vi "Set Description.vi"(8 "error in":errorcluster, 10 "description":string, 11 "data sharing framework custom device in":T1 format="%.0x") -> (0 "error out":errorcluster, 3 "data sharing framework custom deviceout":T1 format="%.0x")   [LabVIEW 2017, in "Data Sharing Framework Custom Device Scripting.lvlib"]
doc: "Writes the <b>description</b> field for the input Data Sharing Framework custom device."
uses:
  Data Sharing Framework Custom Device Scripting.lvlib
  <vilib>/NI Veristand/Custom Device API/Custom Device Item Ref.ctl
  <vilib>/NI VeriStand/Custom Device API/Custom Device API.lvlib
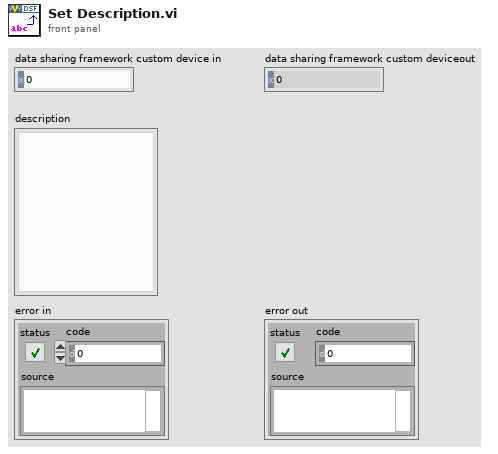
[diagram p1: front panel]
types:
  T1 = typedef "Custom Device API.lvlib/Custom Device Item Ref.ctl" = u64
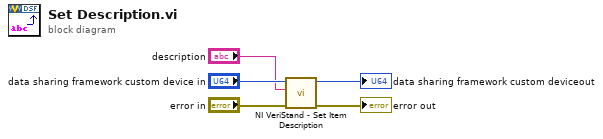
[diagram p0: block diagram]
diagram:
  n1 = call <vilib>:"NI VeriStand - Set Item Description.vi"("error in (no error)"="error in", "Description"="description", "Item Ref in"="data sharing framework custom device in") -> ("error out"=→"error out":errorcluster, "Item Ref out"=→"data sharing framework custom deviceout":T1)  [unwired: 6 in, 1 out]
